vi "Create Msg Queue.vi"(7 "Max Size (-1)":i32=-1, 8 "error in":errorcluster, 9 "Initial Msg Value":variant, 10 "Initial Msg Name":string, 11 "Queue Name":string) -> (0 "error out":errorcluster, 3 "queue out":refnum<queue>)   [LabVIEW 2018, in "EZ Message.lvlib"]
uses:
  EZ Message.lvlib
  Message.ctl
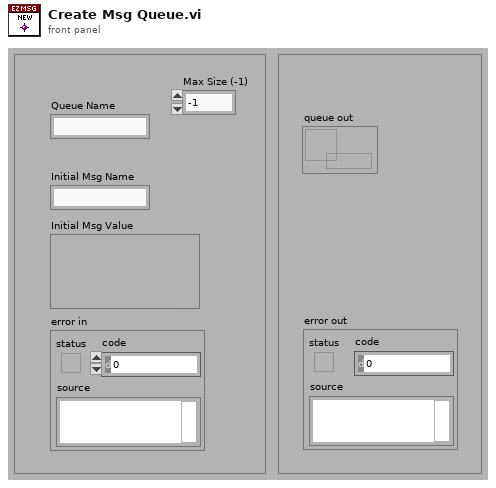
[diagram p1: front panel]
types:
  T1 = typedef "EZ Message.lvlib/Message.ctl" = cluster{"Name":string, "Value":variant}
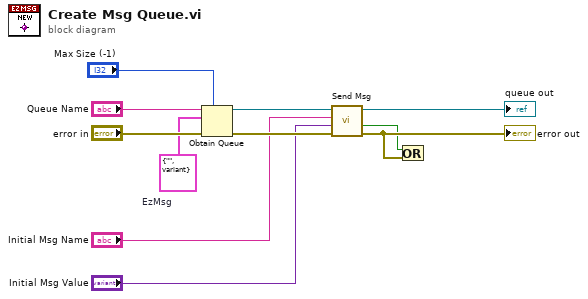
[diagram p0: block diagram]
diagram:
  w4 = T1 {"Name"="", "Value"=variant}  # EzMsg
  n1 = Obtain Queue(max queue size (-1, unlimited)="Max Size (-1)", name (unnamed)="Queue Name", element data type=w4, error in (no error)="error in") -> (queue out=w7:refnum<queue>, error out=w8:errorcluster)  [unwired: 1 in, 1 out]
  n2 = call "Send Msg.vi"("error in"=w8, "Msg Value"="Initial Msg Value", "Msg Name"="Initial Msg Name", "Msg Queue In"=w7) -> ("error out"=w11:errorcluster, "timed out?"=w3:bool, "Msg Queue Out"=→"queue out":refnum<queue>)  [unwired: 4 in, 1 out]
  "error out" <- w11
  n3 = Or(x=w3, y=w11) -> ()  [unwired: 1 out]
